vi "SolarFault.vi"(8 "System Control":T1={"Start"=FALSE, "Stop"=FALSE, "Power System Enable"=FALSE, "SSG Control"=FALSE, "Virtual Inertia"=FALSE, "Manual Current"=FALSE, "Discharge"=FALSE, "Spot Generation"=FALSE, "Charge Control"=FALSE, "Watchdog"=FALSE, "ComAp Fault"=FALSE, "Clear Gen Faults"=FALSE, "Clear PV Faults"=FALSE, "Clear System Faults"=FALSE, "Clear PC Faults"=FALSE, "Clear ES Faults"=FALSE, "Clear Watchdog Faults"=FALSE, "PS V Setpoint"=0.0, "Manual Current"=0.0, "CC V Setpoint"=0.0, "Gen Capacity"=0.0, "Gen Reserve"=0.0, "VI gain P"=0.0, "CC gain P"=0.0, "Nom Hz"=0.0, "Spot Gen Op Value"=50.0, "CC gain I"=0.0, "CC Charge"=100.0, "CC Discharge"=-100.0, "Discharge Current"=-25.0, "Sign Of Life"=FALSE}, 10 "SSG Data":T2, 11 "PV Control":bool) -> (0 "PV Fault":bool, 3 "PV Contactor":bool)   [LabVIEW 2013]
uses:
  <vilib>/ptbypt/NI_PtbyPt.lvlib
  eng/trunk/ni/cRIO Master Files/Controls/SystemControl.ctl
  Controls/FPGAData.ctl
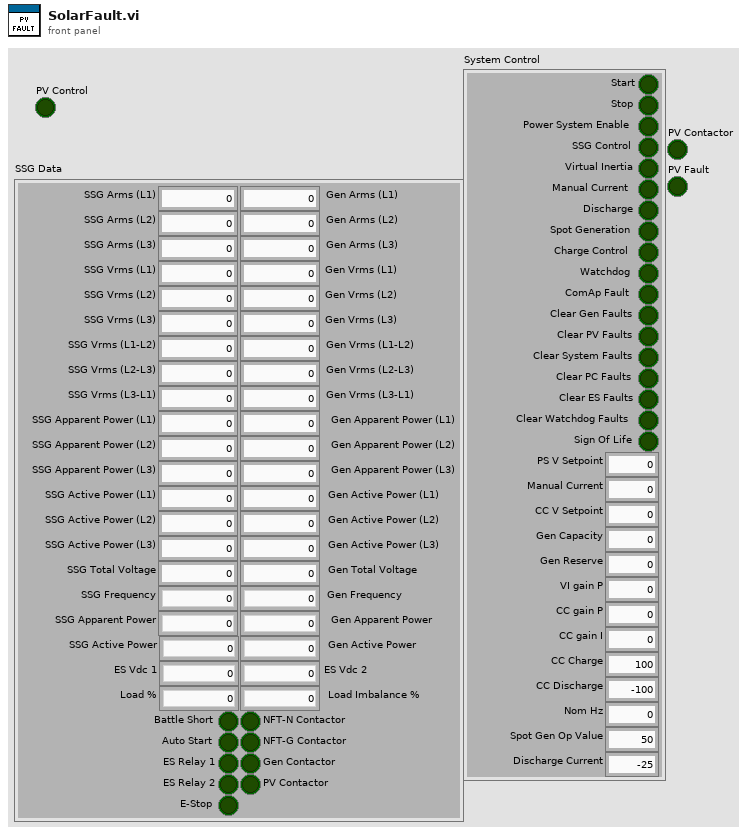
[diagram p1: front panel]
types:
  T1 = typedef "SystemControl.ctl" = cluster{"Start":bool, "Stop":bool, "Power System Enable":bool, "SSG Control":bool, "Virtual Inertia":bool, "Manual Current":bool, "Discharge":bool, "Spot Generation":bool, "Charge Control":bool, "Watchdog":bool, "ComAp Fault":bool, "Clear Gen Faults":bool, "Clear PV Faults":bool, "Clear System Faults":bool, "Clear PC Faults":bool, "Clear ES Faults":bool, "Clear Watchdog Faults":bool, "PS V Setpoint":dbl, "Manual Current":dbl, "CC V Setpoint":dbl, "Gen Capacity":dbl, "Gen Reserve":dbl, "VI gain P":dbl, "CC gain P":dbl, "Nom Hz":dbl, "Spot Gen Op Value":dbl, "CC gain I":dbl, "CC Charge":dbl, "CC Discharge":dbl, "Discharge Current":dbl, "Sign Of Life":bool}
  T2 = typedef "FPGAData.ctl" = cluster{"SSG Frequency":sgl, "SSG Total Voltage":dbl, "SSG Active Power":sgl, "SSG Apparent Power":sgl, "SSG Active Power (L1)":dbl, "SSG Active Power (L2)":dbl, "SSG Active Power (L3)":dbl, "SSG Apparent Power (L1)":dbl, "SSG Apparent Power (L2)":dbl, "SSG Apparent Power (L3)":dbl, "SSG Vrms (L1-L2)":dbl, "SSG Vrms (L2-L3)":dbl, "SSG Vrms (L3-L1)":dbl, "SSG Vrms (L1)":dbl, "SSG Vrms (L2)":dbl, "SSG Vrms (L3)":dbl, "SSG Arms (L1)":dbl, "SSG Arms (L2)":dbl, "SSG Arms (L3)":dbl, "Gen Frequency":sgl, "Gen Total Voltage":dbl, "Gen Active Power":sgl, "Gen Apparent Power":sgl, "Gen Active Power (L1)":dbl, "Gen Active Power (L2)":dbl, "Gen Active Power (L3)":dbl, "Gen Apparent Power (L1)":dbl, "Gen Apparent Power (L2)":dbl, "Gen Apparent Power (L3)":dbl, "Gen Vrms (L1-L2)":dbl, "Gen Vrms (L2-L3)":dbl, "Gen Vrms (L3-L1)":dbl, "Gen Vrms (L1)":dbl, "Gen Vrms (L2)":dbl, "Gen Vrms (L3)":dbl, "Gen Arms (L1)":dbl, "Gen Arms (L2)":dbl, "Gen Arms (L3)":dbl, "ES Vdc 1":sgl, "ES Vdc 2":sgl, "Load %":sgl, "Load Imbalance %":sgl, "E-Stop":bool, "Battle Short":bool, "Auto Start":bool, "Gen Contactor":bool, "ES Relay 1":bool, "ES Relay 2":bool, "NFT-N Contactor":bool, "NFT-G Contactor ":bool, "PV Contactor":bool}
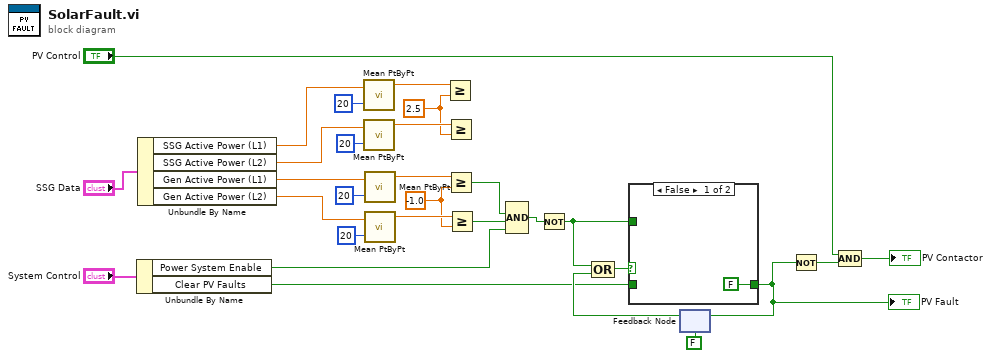
[diagram p0: block diagram]
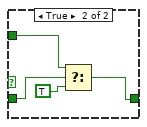
[diagram p2: hidden frame]
diagram:
  w3 = 2.5 ("y")
  w16 = -1.0 ("y")
  n1 = Unbundle By Name("System Control") -> ("Power System Enable"=w23:bool, "Clear PV Faults"=w14:bool)
  n2 = Unbundle By Name("SSG Data") -> ("SSG Active Power (L1)"=w1:dbl, "SSG Active Power (L2)"=w2:dbl, "Gen Active Power (L1)"=w12:dbl, "Gen Active Power (L2)"=w11:dbl)
  n3 = call <vilib>:"Mean PtByPt.vi"("x"=w1, "sample length"=20) -> ("mean"=w5:dbl)  [unwired: 2 in, 1 out]
  n4 = call <vilib>:"Mean PtByPt.vi"("x"=w2, "sample length"=20) -> ("mean"=w4:dbl)  [unwired: 2 in, 1 out]
  n5 = call <vilib>:"Mean PtByPt.vi"("x"=w12, "sample length"=20) -> ("mean"=w18:dbl)  [unwired: 2 in, 1 out]
  n6 = call <vilib>:"Mean PtByPt.vi"("x"=w11, "sample length"=20) -> ("mean"=w17:dbl)  [unwired: 2 in, 1 out]
  n7 = Greater Or Equal?(x=w5, y=w3) -> ()  [unwired: 1 out]
  n8 = Greater Or Equal?(x=w4, y=w3) -> ()  [unwired: 1 out]
  n9 = Greater Or Equal?(x=w18, y=w16) -> (x >= y?=w21:bool)
  n10 = Greater Or Equal?(x=w17, y=w16) -> (x >= y?=w22:bool)
  n11 = Compound Arithmetic op=AND(w21, w22, w23) -> (w15:bool)  [unwired: 1 in]
  n12 = Not(x=w15) -> (.not. x?=w24:bool)
  n13 = feedback #1(FALSE) -> (w25:bool)
  n14 = Compound Arithmetic op=OR(w24, w25) -> (w27:bool)
  n15 = case shown="False" w27 {
    tunnel: [FALSE w31] -> w13
    tunnel: w14 -> [_ w34]
    tunnel: w24 -> [_ w33]
    frame False {
    }
    frame True {
      n16 = Select(t=w33, s=w34, f=TRUE) -> (s? t:f=w31:bool)
    }
  }
  "PV Fault" <- w13
  n17 = feedback-in #1(w13) -> ()
  n18 = Not(x=w13) -> (.not. x?=w9:bool)
  n19 = Compound Arithmetic op=AND("PV Control", w9) -> (→"PV Contactor":bool)
